vi "Write FPGA Setting.vi"(8 "error in (no error)":errorcluster, 10 "FPGA Setting":T1={"Numeric"=0.5, "Combo"="", "String"="", "Boolean"=FALSE} {"Numeric" format="%#_f"}, 11 "FPGA configuration in":refnum<class "FPGA configuration.lvclass">) -> (0 "error out":errorcluster, 3 "FPGA configuration out":refnum<class "FPGA configuration.lvclass">)   [LabVIEW 2025, in "FPGA.lvlib" / "FPGA configuration.lvclass"]
uses:
  FPGA configuration.lvclass
  FPGA Setting.ctl
  FPGA configuration.lvclass/FPGA configuration.ctl
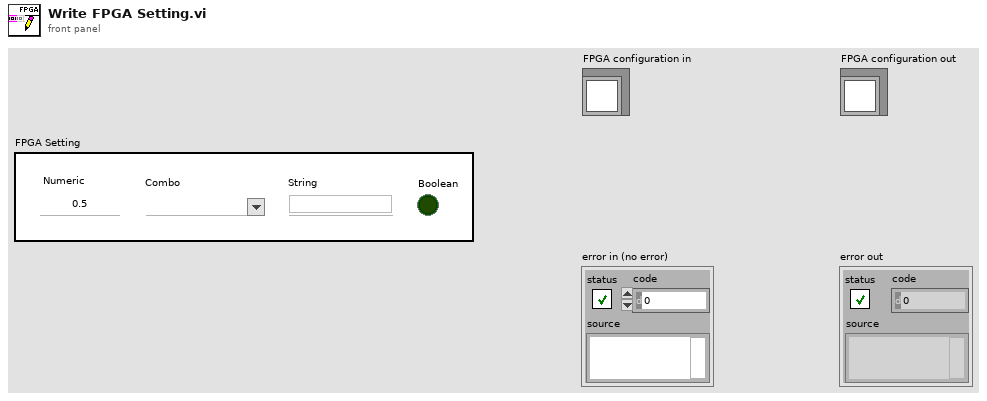
[diagram p1: front panel]
types:
  T1 = typedef "FPGA.lvlib/FPGA configuration.lvclass/FPGA Setting.ctl" = cluster{"Numeric":dbl, "Combo":string, "String":string, "Boolean":bool}
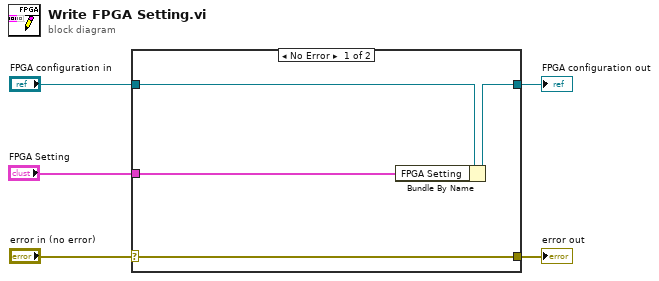
[diagram p0: block diagram]
diagram:
  n1 = case shown="No Error" "error in (no error)" {
    selector: "error in (no error)" -> [w9 w10]
    tunnel: [w9 w10] -> w4
    tunnel: [w7 w11] -> w2
    tunnel: "FPGA configuration in" -> [w8 w11]
    tunnel: "FPGA Setting" -> [w6 _]
    frame No Error {
      n2 = Bundle By Name(cluster=w8, "FPGA Setting"=w6) -> (w7:refnum<class "FPGA configuration.lvclass">)
    }
    frame Error {
    }
  }
  "error out" <- w4
  "FPGA configuration out" <- w2
